vi "Signal FPGA to start acquisition.vi"(8 "error in (no error)":errorcluster, 10 "Logging queue element":T1={"Imaging Protocol"=enum."Live Imaging", "Number of Trials"=0, "Frame Size"=512, "# Averaged frames"=0, "Dwell time (us)"=0.0, "Index of Z-plane"=0, "Timelapse?"=FALSE, "Logging process is active"=FALSE, "Speed logging enabled"=FALSE, "tdms file ref"=refnum, "path"=path "", "Trial Number"=0, "Expected # points acquired"=FALSE, "Manually stopped"=FALSE, "Last trial"=FALSE, "Ch0 data"=[], "Ch1 data"=[], "Image Time"=[], "Continuous Time"=[], "Points acquired"={"Ch0 last trial"=0, "Ch1 last trial"=0, "All trials"=0}, "HW Timings File"=refnum} {"Frame Size" items=["100X100"=100, "128X128"=128, "200X200"=200, "256X256"=256, "512X512"=512, "1024x1024"=1024, "2048x2048"=2048]; "Dwell time (us)" format="%#.6g"}, 11 "FPGA VI Ref":T5) -> (0 "error out":errorcluster, 3 "FPGA VI Reference Out":T5)   [LabVIEW 2017]
uses:
  RIG-SPECIFIC FILES/FPGA Refs/FPGA Ref.ctl
  Typedefs/Logging queue element.ctl
  Typedefs/Imaging Protocols enum.ctl
  Typedefs/Frame Size.ctl
  Typedefs/Acquired points count.ctl
  <vilib>/Utility/error.llb/Error Cluster From Error Code.vi
  <vilib>/rvi/errors/niLvFpgaAdjustHostInterfaceError.vi
  Global Variables/General Globals.vi
  <vilib>/rvi/interface/nirviReadWriteControl/nirviReadWriteControl.xnode
  NiFpgaLv.dll
  <vilib>/rvi/interface/Simulation/niFpgaSimulationCallBeginRW.vi
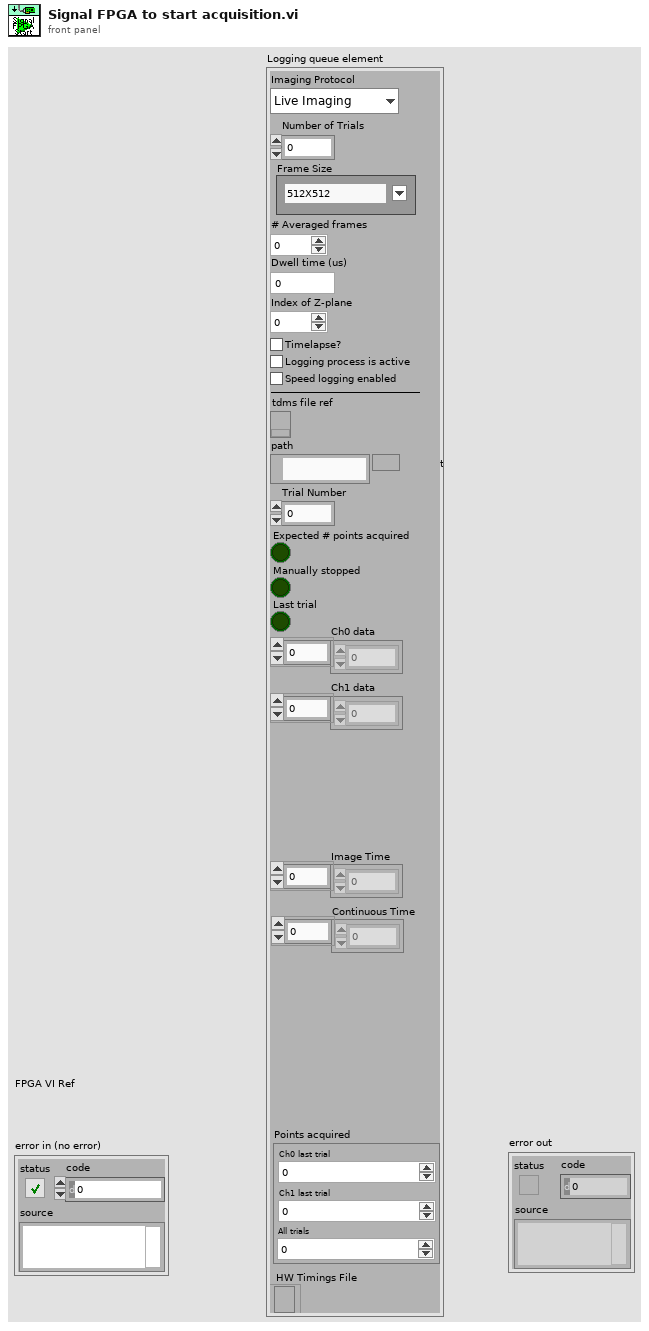
[diagram p1: front panel]
types:
  T1 = typedef "Logging queue element.ctl" = cluster{"Imaging Protocol":T2, "Number of Trials":u16, "Frame Size":T3, "# Averaged frames":u16, "Dwell time (us)":dbl, "Index of Z-plane":i32, "Timelapse?":bool, "Logging process is active":bool, "Speed logging enabled":bool, "tdms file ref":refnum<k34>, "path":path, "Trial Number":i32, "Expected # points acquired":bool, "Manually stopped":bool, "Last trial":bool, "Ch0 data":u32[], "Ch1 data":u32[], "Image Time":u64[], "Continuous Time":u64[], "Points acquired":T4, "HW Timings File":refnum<file>}
  T2 = typedef "Imaging Protocols enum.ctl" = enum16{"AOL Z-Stack", "Motor Z Stack", "Functional Acquisition", "Single Plane Acquisition", "Volume Acquisition", "Live Imaging", "Live Plane Imaging", "Live Volume Imaging"}
  T3 = typedef "Frame Size.ctl" = u16
  T4 = typedef "Acquired points count.ctl" = cluster{"Ch0 last trial":u64, "Ch1 last trial":u64, "All trials":u64}
  T5 = typedef "FPGA Ref.ctl" = refnum<k20>
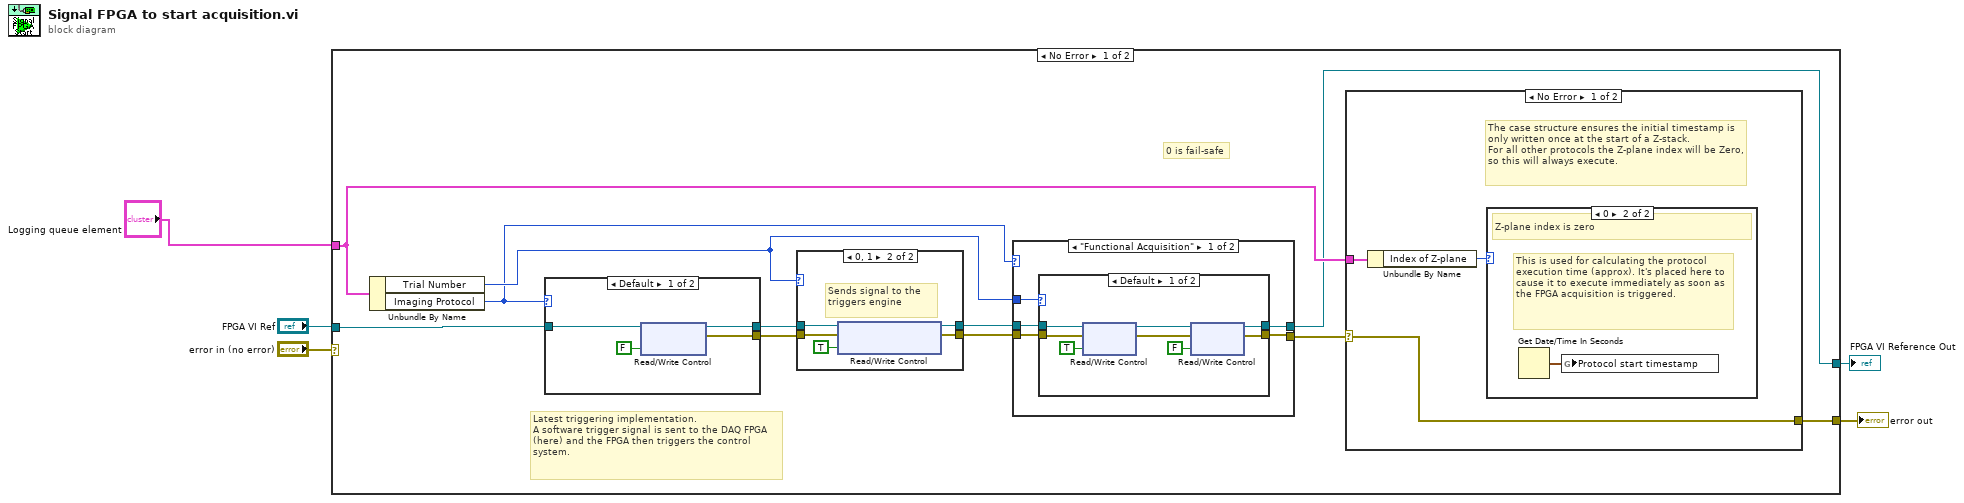
[diagram p0: block diagram]
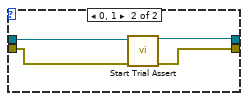
[diagram p2: hidden frame]
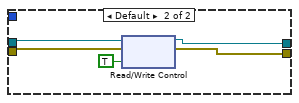
[diagram p3: hidden frame]
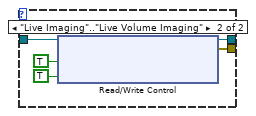
[diagram p7: hidden frame]
diagram:
  n1 = case shown="No Error" "error in (no error)" {
    selector: "error in (no error)" -> [_ w61]
    tunnel: [w15 w61] -> w5
    tunnel: "FPGA VI Ref" -> [w16 w60]
    tunnel: "Logging queue element" -> [w14 _]
    tunnel: [w6 w60] -> w2
    frame No Error {
      # "0 is fail-safe"
      # "Latest triggering implementation.\nA software trigger signal is sent to the DAQ FPGA (here) and the FPGA then triggers the control system."
      n2 = Unbundle By Name(w14) -> ("Trial Number"=w11:i32, "Imaging Protocol"=w8:T2)
      n3 = case shown="Default" w8 {
        tunnel: w16 -> [w53 w59]
        tunnel: [w52 w58] -> w13
        tunnel: [w51 w56] -> w12
        frame Default {
          n4 = xnode "Read/Write Control"("FPGA VI Reference In"=w53, "live_scan"=FALSE) -> ("FPGA VI Reference Out"=w52:T5, "error out"=w51:errorcluster)  [unwired: 1 in]
        }
        frame "Live Imaging".."Live Volume Imaging" {
          n5 = xnode "Read/Write Control"("FPGA VI Reference In"=w59, "live_scan"=TRUE, "live_scan (triggers module)"=TRUE) -> ("FPGA VI Reference Out"=w58:T5, "error out"=w56:errorcluster)  [unwired: 1 in]
        }
      }
      n6 = case shown="0, 1" w11 {
        tunnel: w12 -> [w40 w44]
        tunnel: [w40 w43] -> w9
        tunnel: w13 -> [w39 w42]
        tunnel: [w39 w41] -> w10
        frame Default {
        }
        frame 0, 1 {
          # "Sends signal to the triggers engine"
          n7 = xnode "Read/Write Control"("FPGA VI Reference In"=w42, "error in"=w44, "Experiment start"=TRUE ("start")) -> ("FPGA VI Reference Out"=w41:T5, "error out"=w43:errorcluster)
        }
      }
      n8 = case shown="\"Functional Acquisition\"" w8 {
        tunnel: w10 -> [w20 w37]
        tunnel: w9 -> [w18 w36]
        tunnel: [w19 w35] -> w6
        tunnel: [w17 w34] -> w7
        tunnel: w11 -> [w21 _]
        frame "Functional Acquisition" {
          n9 = case shown="Default" w21 {
            tunnel: w20 -> [w28 w33]
            tunnel: [w25 w31] -> w19
            tunnel: w18 -> [w27 w32]
            tunnel: [w22 w30] -> w17
            frame Default {
              n10 = xnode "Read/Write Control"("FPGA VI Reference In"=w28, "error in"=w27, "start"=TRUE) -> ("FPGA VI Reference Out"=w24:T5, "error out"=w23:errorcluster)
              n11 = xnode "Read/Write Control"("FPGA VI Reference In"=w24, "error in"=w23, "start"=FALSE) -> ("FPGA VI Reference Out"=w25:T5, "error out"=w22:errorcluster)
            }
            frame 0, 1 {
              n12 = call "Start Trial Assert.vi"("error in"=w32, "FPGA VI Ref"=w33) -> ("error out"=w30:errorcluster, "FPGA VI Reference Out"=w31:T5)  [unwired: 8 in]
            }
          }
        }
        frame Default {
          n13 = xnode "Read/Write Control"("FPGA VI Reference In"=w37, "error in"=w36, "start"=TRUE) -> ("FPGA VI Reference Out"=w35:T5, "error out"=w34:errorcluster)
        }
      }
      n14 = case shown="No Error" w7 {
        selector: w7 -> [w48 w50]
        tunnel: [w48 w50] -> w15
        tunnel: w14 -> [w47 _]
        frame No Error {
          # "The case structure ensures the initial timestamp is only written once at the start of a Z-stack.\nFor all other protocols the Z-plane index will be Zero, so this will always execute."
          n15 = Unbundle By Name(w47) -> ("Index of Z-plane"=w46:i32)
          n16 = case shown="0" w46 {
            frame Default {
              # "Z-plane index is other than zero"
            }
            frame 0 {
              # "This is used for calculating the protocol execution time (approx). It's placed here to cause it to execute immediately as soon as the FPGA acquisition is triggered."
              # "Z-plane index is zero"
              n17 = Get Date/Time In Seconds() -> (seconds since 1Jan1904=w49:timestamp)
              n18 = global write "General Globals.vi" "Protocol start timestamp"(w49) -> ()
            }
          }
        }
        frame Error {
        }
      }
    }
    frame Error {
    }
  }
  "error out" <- w5
  "FPGA VI Reference Out" <- w2
